vi "Deadband.vi"(1 "Deadband":dbl=0.02, 3 "Value":dbl) -> (0 "Output":dbl)   [LabVIEW 2018]
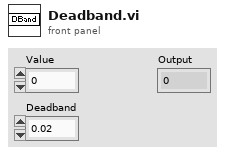
[diagram p1: front panel]
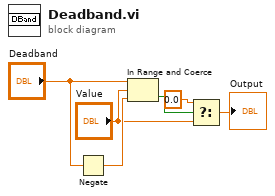
[diagram p0: block diagram]
diagram:
  n1 = Negate(x="Deadband") -> (-x=w4:dbl)
  n2 = In Range and Coerce(upper limit="Deadband", x="Value", lower limit=w4) -> (In Range?=w6:bool)  [unwired: 1 out]
  n3 = Select(t=0.0, s=w6, f="Value") -> (s? t:f=→"Output":dbl)
